vi "OSICS_Get_Enable_Disable.vi"(7 "OSICS slot":i32=1 min=1 max=8 step=1, 8 "error in":errorcluster, 11 "VISA IN":refnum<visa-resource-name>) -> (0 "error out":errorcluster, 2 "Enable/Disable (False:Disabled)":bool=TRUE, 3 "VISA OUT":refnum<visa-resource-name>, 5 "ERR":i32)   [LabVIEW 2014, in "OSICS_LIB.lvlib"]
doc: "This Vi enables/disables the output of OSICS modules."
uses:
  OSICS_LIB.lvlib
  <vilib>/regexp/Match Regular Expression.xnode
panel:
  # "BASIC Function to  Get Enable/Disable state of the OSICS"
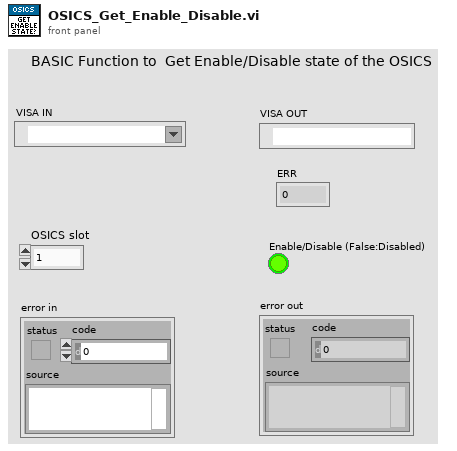
[diagram p1: front panel]
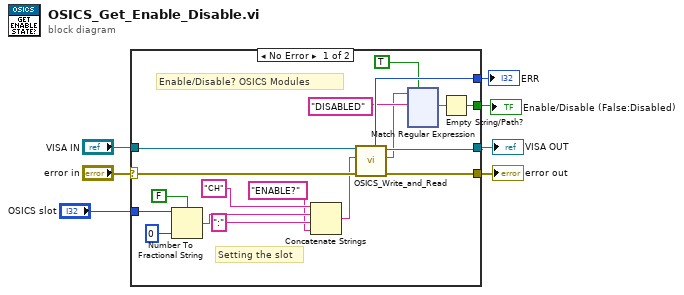
[diagram p0: block diagram]
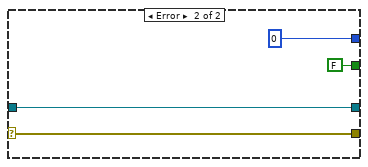
[diagram p2: hidden frame]
diagram:
  n1 = case shown="No Error" "error in" {
    selector: "error in" -> [w22 w139]
    tunnel: "VISA IN" -> [w23 w140]
    tunnel: [w25 w140] -> w6
    tunnel: [w24 w139] -> w5
    tunnel: [w13 0 ("ERR")] -> w3
    tunnel: "OSICS slot" -> [w20 _]
    tunnel: [w11 FALSE] -> w1
    frame No Error {
      # "Setting the slot"
      # "Enable/Disable? OSICS Modules"
      n2 = Number To Fractional String(use system decimal point (T)=FALSE, number=w20, precision (6)=i16 0) -> (F-format string=w18:string)  [unwired: 1 in]
      n3 = Concatenate Strings("CH" ("string"), w18, ":" ("string"), "ENABLE?") -> (w16:string)
      n4 = call "OSICS_Write_and_Read.vi"("error in (no error)"=w22, "String to Send"=w16, "VISA IN"=w23) -> ("error out"=w24:errorcluster, "Message Available"=w9:string, "VISA OUT"=w25:refnum<visa-resource-name>, "ERR"=w13:i32)  [unwired: 5 in]
      n5 = xnode "Match Regular Expression"("input string"=w9, "regular expression"="DISABLED", "ignore case? (F)"=TRUE) -> ("whole match"=w12:string)  [unwired: 3 in, 4 out]
      n6 = Empty String/Path?(string/path=w12) -> (empty?=w11:bool)
    }
    frame Error {
    }
  }
  "error out" <- w5
  "VISA OUT" <- w6
  "ERR" <- w3
  "Enable/Disable (False:Disabled)" <- w1
